vi "模拟输入_软件按需单点.vi"() -> ()   [LabVIEW 2013]
doc: "This example demonstrates how to measure voltage using a software timer."
uses:
  <userlib>/ArtDAQ/_SubVI/ArtDAQ_CreateAIVoltageChan.vi
  <userlib>/ArtDAQ/_SubVI/ArtDAQ_Read Analog DBL NChan 1Samp.vi
panel:
  out "数据":dbl[](array[numeric])
  in  "定时 (ms)":u32=100
  in  "Stop":bool
  in  "接线端配置":i32(ring)=-1 items=["默认"=-1, "单端"=10083, "非参考单端"=10078, "差分"=10106, "伪差分"=12529]
  in  "最小值(V)":dbl=-10.0 format="%#_13g"
  in  "最大值(V)":dbl=10.0 format="%#_13g"
  in  "物理通道":string(combo)="Dev1/ai0"
  out "错误":errorcluster
  # "通道属性"
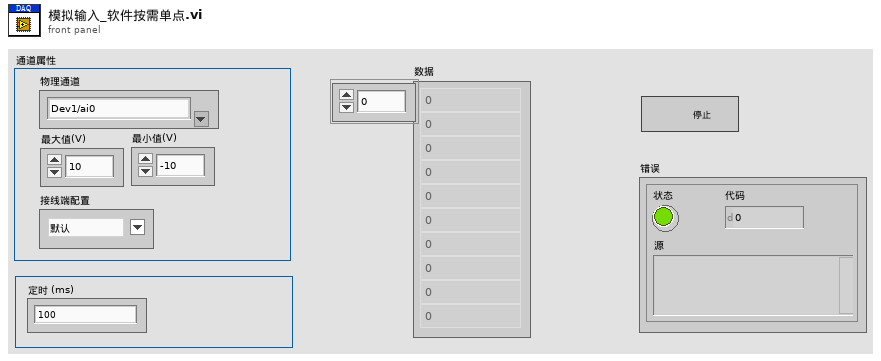
[diagram p1: front panel]
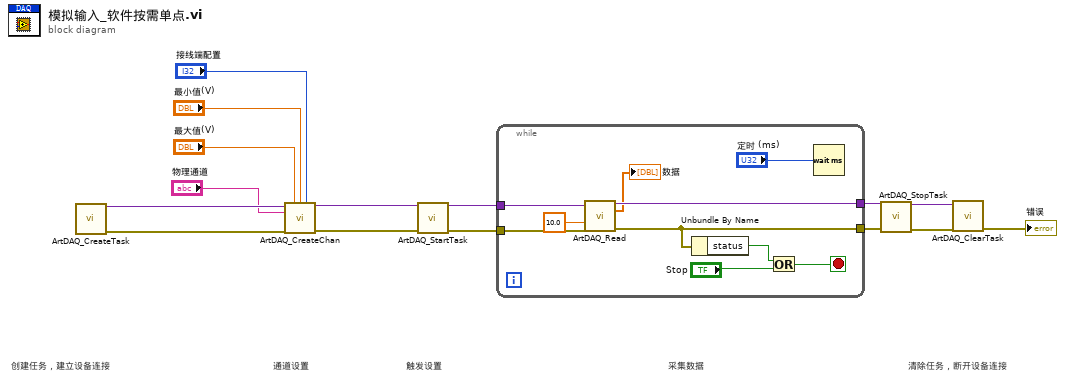
[diagram p0: block diagram]
diagram:
  # "清除任务，断开设备连接"
  # "采集数据"
  # "触发设置"
  # "通道设置"
  # "创建任务，建立设备连接"
  n1 = call <userlib>:"ArtDAQ_CreateTask.vi"() -> ("任务句柄"=w8:variant, "错误输出"=w15:errorcluster)  [unwired: 14 in]
  n2 = call-poly <userlib>:"ArtDAQ_CreateChan.vi"("任务句柄"=w8, "最大值"="最大值(V)", "最小值"="最小值(V)", "接线端配置"="接线端配置", "物理通道"="物理通道", "错误输入"=w15) -> ("任务句柄"=w2:variant, "错误输出"=w1:errorcluster)  [unwired: 8 in]
  n3 = call <userlib>:"ArtDAQ_StartTask.vi"("任务句柄"=w2, "错误输入"=w1) -> ("任务句柄"=w10:variant, "错误输出"=w9:errorcluster)  [unwired: 12 in]
  n4 = while {
    tunnel: w10 -> [w25]
    tunnel: w9 -> [w24]
    tunnel: [w22] -> w7
    tunnel: [w21] -> w6
    stop <- w19 stop-if-true
    n5 = call-poly <userlib>:"ArtDAQ_Read.vi"("任务句柄"=w25, "超时s"=10.0 ("Timeout"), "错误输入"=w24) -> ("任务句柄"=w22:variant, "数据"=→"数据":dbl[], "错误输出"=w21:errorcluster)  [unwired: 10 in]
    n6 = Unbundle By Name(w21) -> ("status"=w20:bool)
    n7 = Or(x=w20, y="Stop") -> (x .or. y?=w19:bool)
    n8 = Wait (ms)(milliseconds to wait="定时 (ms)") -> ()  [unwired: 1 out]
  }
  n9 = call <userlib>:"ArtDAQ_StopTask.vi"("任务句柄"=w7, "错误输入"=w6) -> ("任务句柄"=w5:variant, "错误输出"=w4:errorcluster)  [unwired: 12 in]
  n10 = call <userlib>:"ArtDAQ_ClearTask.vi"("任务句柄"=w5, "错误输入"=w4) -> ("错误输出"=→"错误":errorcluster)  [unwired: 13 in]
